vi "核查数据编码整合输出.vi"(6 "字段结束":bool=TRUE, 7 "数据标识":string="N", 8 "数据类型":string(combo)="-Rtd=", 9 "污染物编码":string, 10 "数据精度":i32=6, 11 "数据值":string) -> (0 "编码输出":string)   [LabVIEW 2016, in "数据传输系统-06.lvlib"]
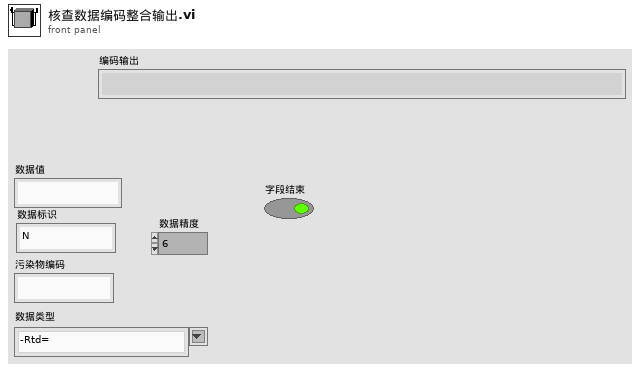
[diagram p1: front panel]
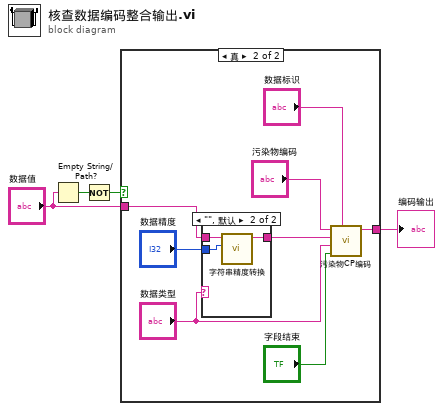
[diagram p0: block diagram]
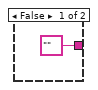
[diagram p2: hidden frame]
diagram:
  n1 = Empty String/Path?(string/path="数据值") -> (empty?=w2:bool)
  n2 = Not(x=w2) -> (.not. x?=w4:bool)
  n3 = case shown="真" w4 {
    tunnel: ["" ("编码输出") w13] -> w1
    tunnel: "数据值" -> [_ w12]
    frame False {
    }
    frame True {
      n4 = case shown="\"\", 默认" "数据类型" {
        tunnel: w12 -> [w14 w17]
        tunnel: [w14 w16] -> w11
        tunnel: "数据精度" -> [_ w15]
        frame "-WaterTime=" {
        }
        frame "", Default {
          n5 = call "字符串精度转换.vi"("数据精度"=w15, "输入字符串"=w17) -> ("输出字符串"=w16:string)  [unwired: 8 in, 1 out]
        }
      }
      n6 = call "污染物CP编码.vi"("字符串"="数据标识", "字段结束"="字段结束", "数据类型"="数据类型", "污染物浓度"=w11, "污染物编码"="污染物编码") -> ("编码输出"=w13:string)  [unwired: 5 in]
    }
  }
  "编码输出" <- w1
